vi "Deprecated.vi"(8 "error in (no error)":errorcluster, 11 "Value in":refnum<class "Value.lvclass">) -> (0 "error out":errorcluster, 3 "Value out":refnum<class "Value.lvclass">)   [LabVIEW 2020, in "Promises.lvlib" / "Value.lvclass"]
uses:
  Value.lvclass
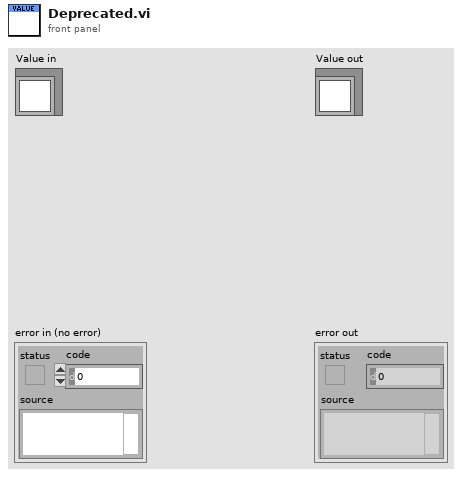
[diagram p1: front panel]
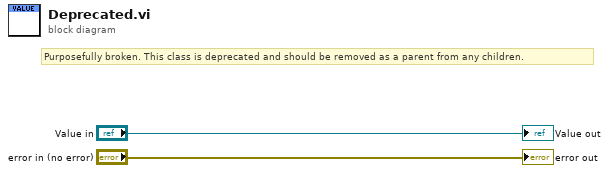
[diagram p0: block diagram]
diagram:
  # "Purposefully broken. This class is deprecated and should be removed as a parent from any children."
  "error out" <- "error in (no error)"
  "Value out" <- "Value in"
